vi "Compression with PCA.vi"() -> ()   [LabVIEW 2023]
doc: "This example shows the application of principal component analysis (PCA) in image compression.\n\nYou can consider each row of the image as a time series and the whole image as a multivariate time series. After applying PCA, the correlation among the rows of the image is reduced. Only a few rows of the resulting principal component scores contain significant information. By keeping only the rows with important information, you can reduce the dimensionality of the image and retain important information of the image. \n\nThis example uses the TSA Principal Component Analysis VI to compute principal component scores of an image and reconstruct the image with only part of the principal component scores that contain significant or useful values.\n\n<b>Instructions:</b>\n1) Run this VI.\n2) Change the number of rows to keep principal component scores with significant information and observe the PSNR of the image."
uses:
  Images/_Images.ctl
  <vilib>/Analysis/baseanly.llb/Real A x B.vi
  <vilib>/addons/Time Series Analysis/Statistical Analysis.llb/TSA Principal Component Analysis (Array).vi
  <vilib>/Analysis/Matrix/Numeric/Conversions/Matrix To Array - RM.vi
  <vilib>/addons/_Advanced Signal Processing/NI_AdvSigProcTSA.lvlib
  <vilib>/Analysis/NI_AALBase.lvlib
  <vilib>/Analysis/Matrix/NI_Matrix.lvlib
  <vilib>/vision/NI_Vision_Development_Module.lvlib
panel:
  out "Maximal Diff":sgl
  out "Minimal Diff":sgl
  in  "Ratio":i32(slide)=5 min=1 max=100 step=1 scale=1.0..25.0
  out "Weights":dbl[][](graph)
  out "Weights stored":dbl[][](graph)
  out "Scores strored":dbl[][](graph)
  out "Difference":T1(plugin-control)
  out "Reconstructed Image":T1(plugin-control)
  out "Original Image":T1(plugin-control)
  in  "Image":T2=enum."Stepwedge3"
  out "Number of rows to keep":i32
  out "PSNR (dB)":dbl
  out "Scores":dbl[][](graph)
  # "Image Compression and the Principal Component Analysis"
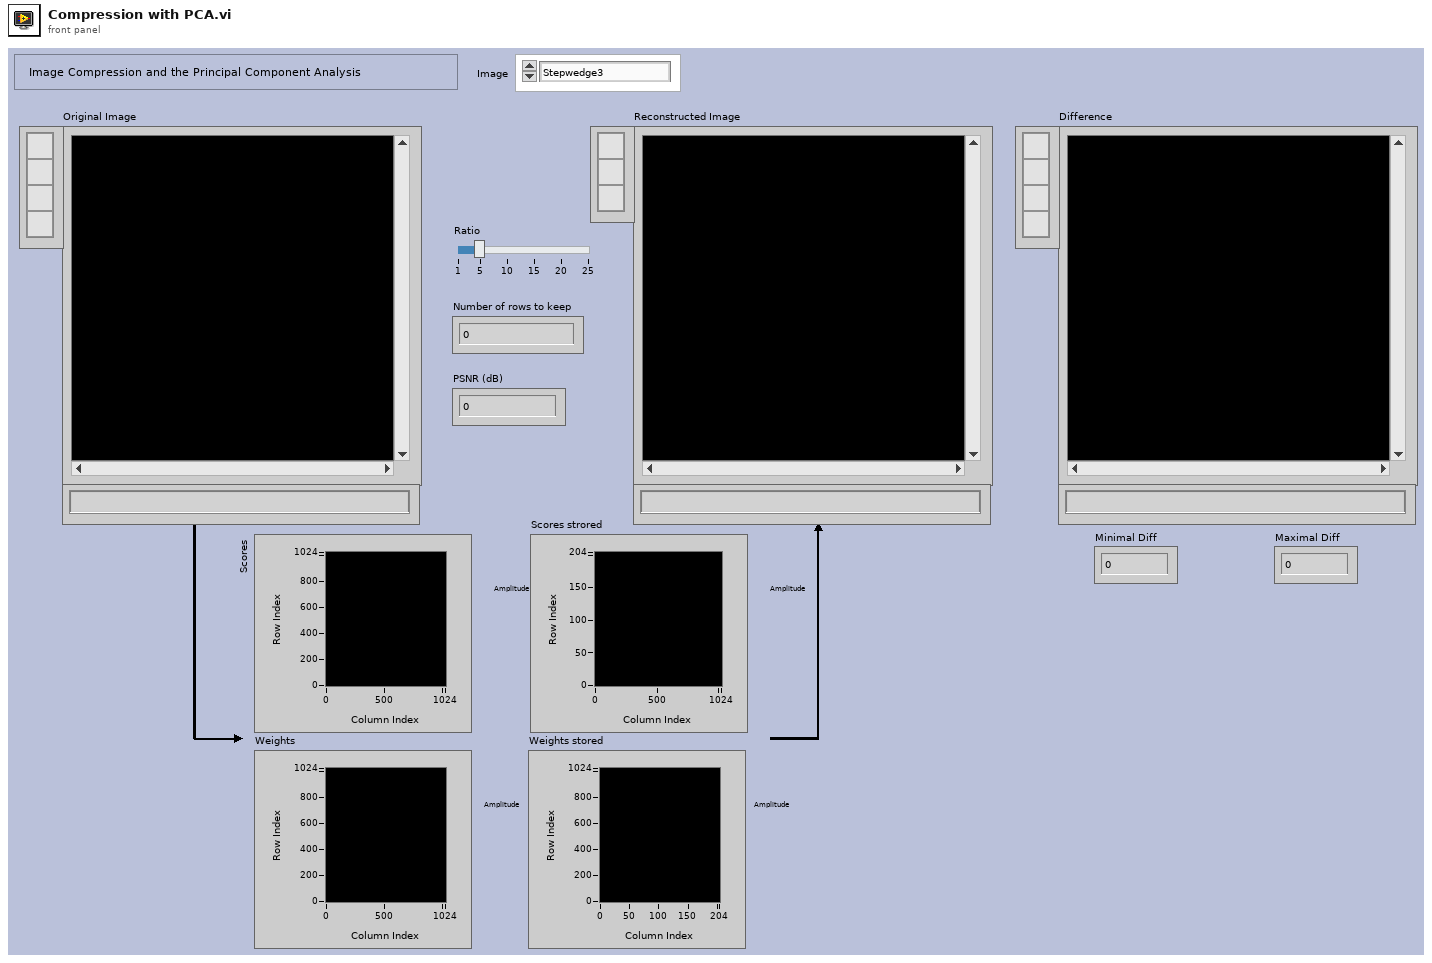
[diagram p1: front panel]
types:
  T1 = typedef "IMAQ Image.ctl" = refnum<image>
  T2 = typedef "_Images.ctl" = enum16{"Balls2", "Battery1", "Battery2", "Connector1", "Subwoofer1", "Subwoofer2", "Subwoofer3", "Subwoofer4", "Hase1", "Lamp1", "Lamp2", "Mouse1", "PhotoLens1", "Po1", "PowerSupply1", "Router", "--- Step Wedges ---", "Stepwedge1", "Stepwedge2", "Stepwedge3", "--- Fusion ---", "Fusion160kV", "Fusion2-120kV", "Fusion2-320kV", "Fusion300kV", "FusionPart1-120kV", "FusionPart1-180kV", "--- PART 01 ---", "Part1", "Part2", "Part3", "Part4", "Part5", "Part6", "Part7", "Part8", "--- Different Integrations ---", "Step2737-02Int", "Step2737-04Int", "Step2737-08Int", "Step2737-16Int", "Step2737-32Int", "Step2737-64Int"}
  T3 = typedef "Image Type" = u32
  T4 = typedef "NI_Matrix.lvlib/RealMatrix.ctl" = dbl[][]
  T5 = cluster{"histogram":u32[], "Minimal Value":sgl, "Maximal Value":sgl, "Starting Value":sgl, "Interval Width":sgl, "Mean Value":sgl, "Standard  Variation":sgl, "Area (pixels)":i32}
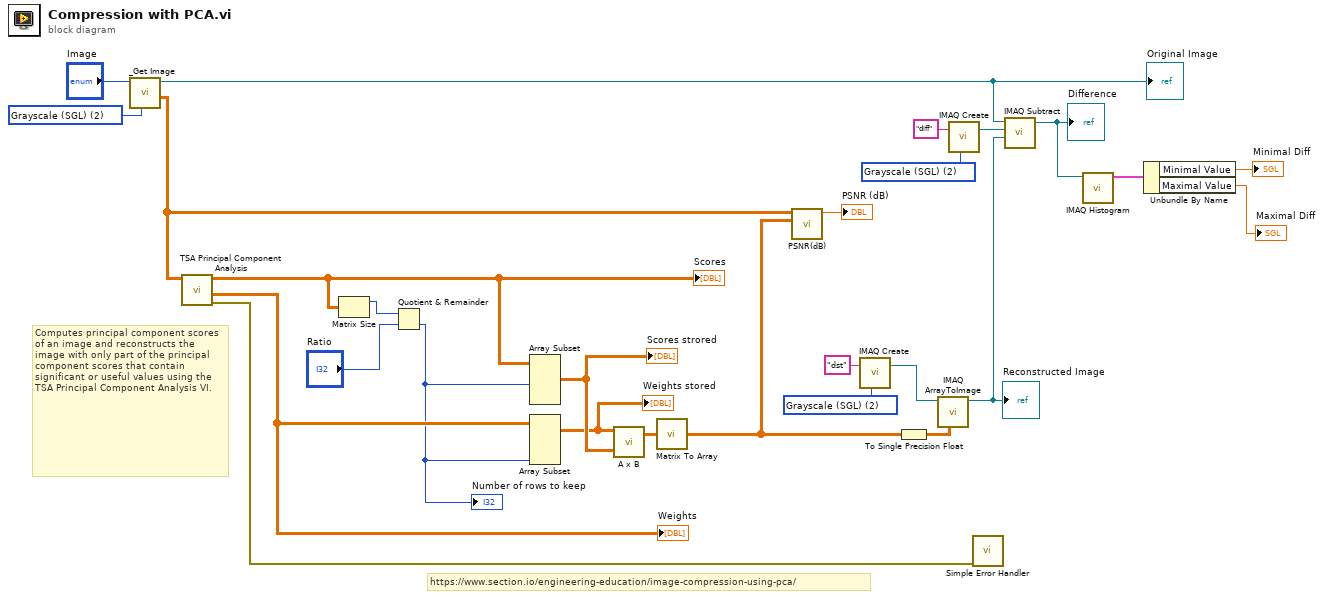
[diagram p0: block diagram]
diagram:
  w19 = T3 2 items=["Grayscale (U8)", "Grayscale (I16)", "Grayscale (SGL)", "Complex (CSG)", "RGB (U32)", "HSL (U32)", "RGB (U64)", "Grayscale (U16)"] ("Image Type")
  w21 = T3 2 items=["Grayscale (U8)", "Grayscale (I16)", "Grayscale (SGL)", "Complex (CSG)", "RGB (U32)", "HSL (U32)", "RGB (U64)", "Grayscale (U16)"] ("Image Type (U16)")
  w23 = T3 2 items=["Grayscale (U8)", "Grayscale (I16)", "Grayscale (SGL)", "Complex (CSG)", "RGB (U32)", "HSL (U32)", "RGB (U64)", "Grayscale (U16)"] ("Image Type")
  # "https://www.section.io/engineering-education/image-compression-using-pca/"
  # "Computes principal component scores of an image and reconstructs the image with only part of the principal component scores that contain significant or useful values using the TSA Principal Component Analysis VI."
  n1 = call "_Get Image.vi"("Image Type (U16)"=w21, "Image"="Image") -> ("Image Pixels (Float)"=w25:dbl[][], "Image Out"=w18:T1)  [unwired: 6 in, 2 out]
  "Original Image" <- w18
  n2 = call-poly <vilib>:"TSA Principal Component Analysis.vi"("Xt"=w25) -> ("error out"=w27:errorcluster, "weights"=w9:dbl[][], "Xt out"=w10:dbl[][])  [unwired: 2 in, 6 out]
  "Scores" <- w10
  "Weights" <- w9
  n3 = Matrix Size(0:w10) -> (1:w8:i32)  [unwired: 1 out]
  n4 = Quotient & Remainder(x=w8, y="Ratio") -> (floor(x/y)=w6:i32)  [unwired: 1 out]
  "Number of rows to keep" <- w6
  n5 = Array Subset(array=w10, length (row)=w6) -> (w12:dbl[][])  [unwired: 3 in]
  "Scores strored" <- w12
  n6 = Array Subset(array=w9, length (col)=w6) -> (w11:dbl[][])  [unwired: 3 in]
  "Weights stored" <- w11
  n7 = call-poly <vilib>:"A x B.vi"("B"=w12, "A"=w11) -> ("A x B"=w15:T4)  [unwired: 1 out]
  n8 = call-poly <vilib>:"Matrix To Array.vi"("Real Matrix"=w15) -> ("Real 2D Array"=w14:dbl[][])
  n9 = call "PSNR(dB).vi"("Image Pixels (Float) 2"=w14, "Image Pixels (Float) 1"=w25) -> ("PSNR (dB)"=→"PSNR (dB)":dbl)  [unwired: 5 in, 4 out]
  n10 = call "IMAQ Create"("Image Name"="dst", "Image Type"=w23) -> ("New Image"=w22:T1)  [unwired: 3 in, 1 out]
  n11 = To Single Precision Float(number=w14) -> (single precision float=w1:sgl[][])
  n12 = call "IMAQ ArrayToImage"("Image Pixels (Float)"=w1, "Image"=w22) -> ("Image Out"=w13:T1)  [unwired: 8 in, 1 out]
  "Reconstructed Image" <- w13
  n13 = call "IMAQ Create"("Image Name"="diff", "Image Type"=w19) -> ("New Image"=w17:T1)  [unwired: 3 in, 1 out]
  n14 = call <vilib>:"Simple Error Handler.vi"("error in (no error)"=w27) -> ()  [unwired: 1 in, 8 out]
  n15 = call "IMAQ Subtract"("Image Src A"=w18, "Image Dst"=w17, "Image Src B"=w13) -> ("Image Dst Out"=w5:T1)  [unwired: 4 in, 1 out]
  "Difference" <- w5
  n16 = call "IMAQ Histogram"("Image"=w5) -> ("Histogram Report"=w4:T5)  [unwired: 9 in, 1 out]
  n17 = Unbundle By Name(w4) -> ("Minimal Value"=→"Minimal Diff":sgl, "Maximal Value"=→"Maximal Diff":sgl)
